vi "Temp_QCM_MKS_SNRaman.vi"() -> ()   [LabVIEW 2013]
doc: "This example demonstrates temperature control and monitoring.\n\nNote:\nBefore start this VI is it necessary:\n\n- preconfigure some specific parameters that are not supported by this driver (e.g. PV-I/O Type, Linearization type, Alarm Input Values... ) by Quick Codes, or by Eurotherm iTools or by instrument front panel controls\n- enter correct VISA Resource Descriptor, Device Address and Baud Rate into front-panel controls"
uses:
  LabVIEW Drivers for DVS instruments/_mks/common/mks pressure units.ctl
  LabVIEW Drivers for DVS instruments/_mks/common/mks status.ctl
  LabVIEW Drivers for DVS instruments/_mks/common/mks status control mode.ctl
  LabVIEW Drivers for DVS instruments/_mks/common/mks status learning mode.ctl
  LabVIEW Drivers for DVS instruments/_mks/common/mks status selection mode.ctl
  LabVIEW Drivers for DVS instruments/_mks/common/mks control direction.ctl
  LabVIEW Drivers for DVS instruments/_mks/common/mks setup communication mode.ctl
  LabVIEW Drivers for DVS instruments/_mks/common/mks setup termination character.ctl
  LabVIEW Drivers for DVS instruments/_mks/common/mks setpoint type.ctl
  LabVIEW Drivers for DVS instruments/_mks/common/mks control type.ctl
  <vilib>/Utility/file.llb/Write To Spreadsheet File (string).vi
  SpectraWiz_LV82_rev04Oct10-1chan-free.llb.llb/StellarNet SpectraWiz Globals.vi
  <instrlib>/Eurotherm 32xx Series/Eurotherm 32xx Series.lvlib
panel:
  in  "Stop SpectraNet Raman":bool
  in  "stop":bool
  in  "Tab Control":T1(tab)
  in  "Add comments to the data file here and click outside the comment box to submit.\nThe time at which comments are submitted is saved in the data file.":string
  out "New ALARM !":bool
  in  "Acknowledge All Alarms":bool
  in  "Controller  Mode":u8(ring) items=["Auto", "Manual"]
  in  "Temp Setpoint (C)":i16(slide)=25 min=0 max=1300 scale=0.0..500.0
  out "Temperature (C)":sgl
  out "Process Value - Chart":sgl(graph)
  in  "Keylock":u8(ring) items=["None", "All", "Edit", "mod", "mAn", "Stby", "tmr"]
  out "Alarm Output":bool
  in  "Alarm \nNumber (1)":u16=1 min=1 max=4
  out "Freq and Resistance Graph":T2(graph)
  out "pressure units 3":T3
  out "Waveform Chart 2":dbl(graph)
  out "status 2":T4
  out "Pressure 2":dbl
  in  "Control direction 3":T8
  in  "Setpoint 2":dbl(knob) min=0.0 max=100.0 scale=0.0..100.0
  out "Control direction 4":T8
  in  "Tab Control 2":T9(tab)=enum."Controls"
  in  "Channel to monitor":i8=1 min=1 max=1
  out "?":T10(graph)
  in  "Use Dark":bool
  in  "Channel":u8=1 min=1 max=1
  in  "Operating Parameters":T11(array[cluster]) {"Digitizer Clock Rate Setting" min=1 max=3; "Optical Smoothing Level" min=0 max=4 step=1; "Number of Scans to Average" min=1 max=10000 step=1}
  in  "Take Dark":bool
  in  "Take Reference":bool
  in  "Mode Selection":u16(ring) items=["Scope Mode", "Absorbance Mode", "Transmission Mode", "Radiometer Mode"]
  in  "View Data File":bool
  in  "Open Data File":bool
  out "?":T10(graph)
  in  "Reset Coefficients":bool
  in  "Drift Correct":bool
  in  "View Snapshot":bool
  in  "Take Snapshot":bool
  out "Number of Channels:":i32
  in  "Clear History":bool
  out "?":T10(graph)
  in  "Create and Log to Time Series Log File":bool
  out "ChartView":T12(graph)
  out "Cursor Indices":i32[](array[numeric])
  out "Data File":cluster{dbl[], dbl[]}
  out "Error Out":errorcluster
  out "Time [s]":dbl format="%.2f"
  # "Configuring Instrument\n \nPlease Wait......\n\nChart will update in 20 sec"
  # "Instructions:\n\nMake sure all instruments are plugged into the correct ports, the correct port numbers are set, and all instruments are turned on. \n\nTo begin, click the RUN arrow on the toolbar, and wait 20 seconds for instruments to begin recording.\n\nTo end, click \"END DATA LOGGING\" and \"Stop Spectra Raman\". DO NOT press the STOP button on the toolbar."
  # "© 2005-2010 StellarNet, Inc.,  All Right Reserved"
  # "``"
  # "© 2005-2013 StellarNet, Inc.,  All Right Reserved"
  # "© 2005-2010 StellarNet, Inc.,  All Right Reserved"
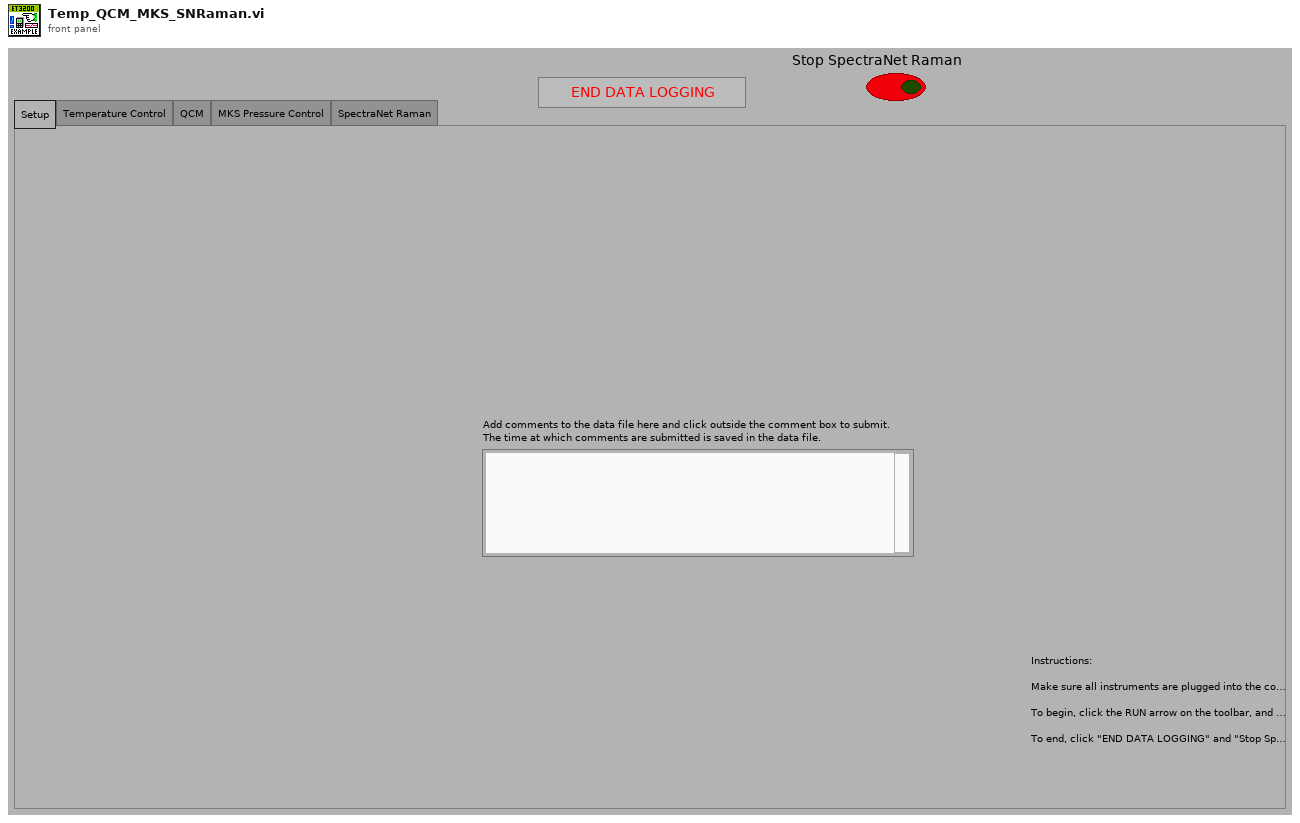
[diagram p1: front panel]
types:
  T1 = enum32{"Setup", "Temperature Control", "QCM", "MKS Pressure Control", "SpectraNet Raman"}
  T2 = cluster{"XY chart data":cluster{"x":dbl, "y":dbl}[]}[]
  T3 = typedef "mks pressure units.ctl" = enum16{"Torr", "mTorr", "mbar", "ubar", "kPa", "Pa", "cmH2O", "inH2O"}
  T4 = typedef "mks status.ctl" = cluster{"control mode":T5, "learning mode":T6, "selection mode":T7}
  T5 = typedef "mks status control mode.ctl" = enum16{"local", "remote"}
  T6 = typedef "mks status learning mode.ctl" = enum16{"not learning", "learning system", "learning valve"}
  T7 = typedef "mks status selection mode.ctl" = enum16{"open", "close", "stop", "setpoint A", "setpoint B", "setpoint C", "setpoint D", "setpoint E", "analog setpoint"}
  T8 = typedef "mks control direction.ctl" = enum16{"direct", "reverse"}
  T9 = enum32{"Graphical Display", "Controls", "Time Series"}
  T10 = cluster{"Spectrometer Wavelengths":dbl[], dbl[]}[]
  T11 = cluster{"Integration Time (ms)":i32, "Number of Scans to Average":i32, "Optical Smoothing Level":i32, "Digitizer Clock Rate Setting":i32, "Temp  Compensation ":bool}[]
  T12 = cluster{"Cursor Y":dbl, "Cursor Y":dbl, "Cursor Y":dbl}
  T13 = typedef "mks setup termination character.ctl" = enum16{"CRLF", "CR"}
  T14 = typedef "mks setup communication mode.ctl" = enum16{"8 databits no parity", "7 databits even parity"}
  T15 = cluster{"Cursor Y":dbl, "Cursor Y":dbl, "Cursor Y":dbl}[]
  T16 = cluster{"Coefficients":ext[], "Wavelengths":dbl[]}[]
  T17 = cluster{"[0]":dbl, "[1]":dbl, "[2]":dbl, "[3]":dbl, "[4]":dbl, "[5]":dbl, "[6]":dbl, "[7]":dbl, "[8]":dbl}
  T18 = cluster{"Minimum":dbl, "Maximum":dbl, "Increment":dbl, "Minor Incr":dbl, "Start":dbl}
  T19 = cluster{"Integration Time (ms)":i32, "Number of Scans to Average":i32, "Optical Smoothing Level":i32, "Digitizer Clock Rate Setting":i32, "Temp  Compensation ":bool}
  T20 = typedef "mks control type.ctl" = enum16{"Self-Tuning", "PID"}
  T21 = typedef "mks setpoint type.ctl" = enum16{"position", "pressure"}
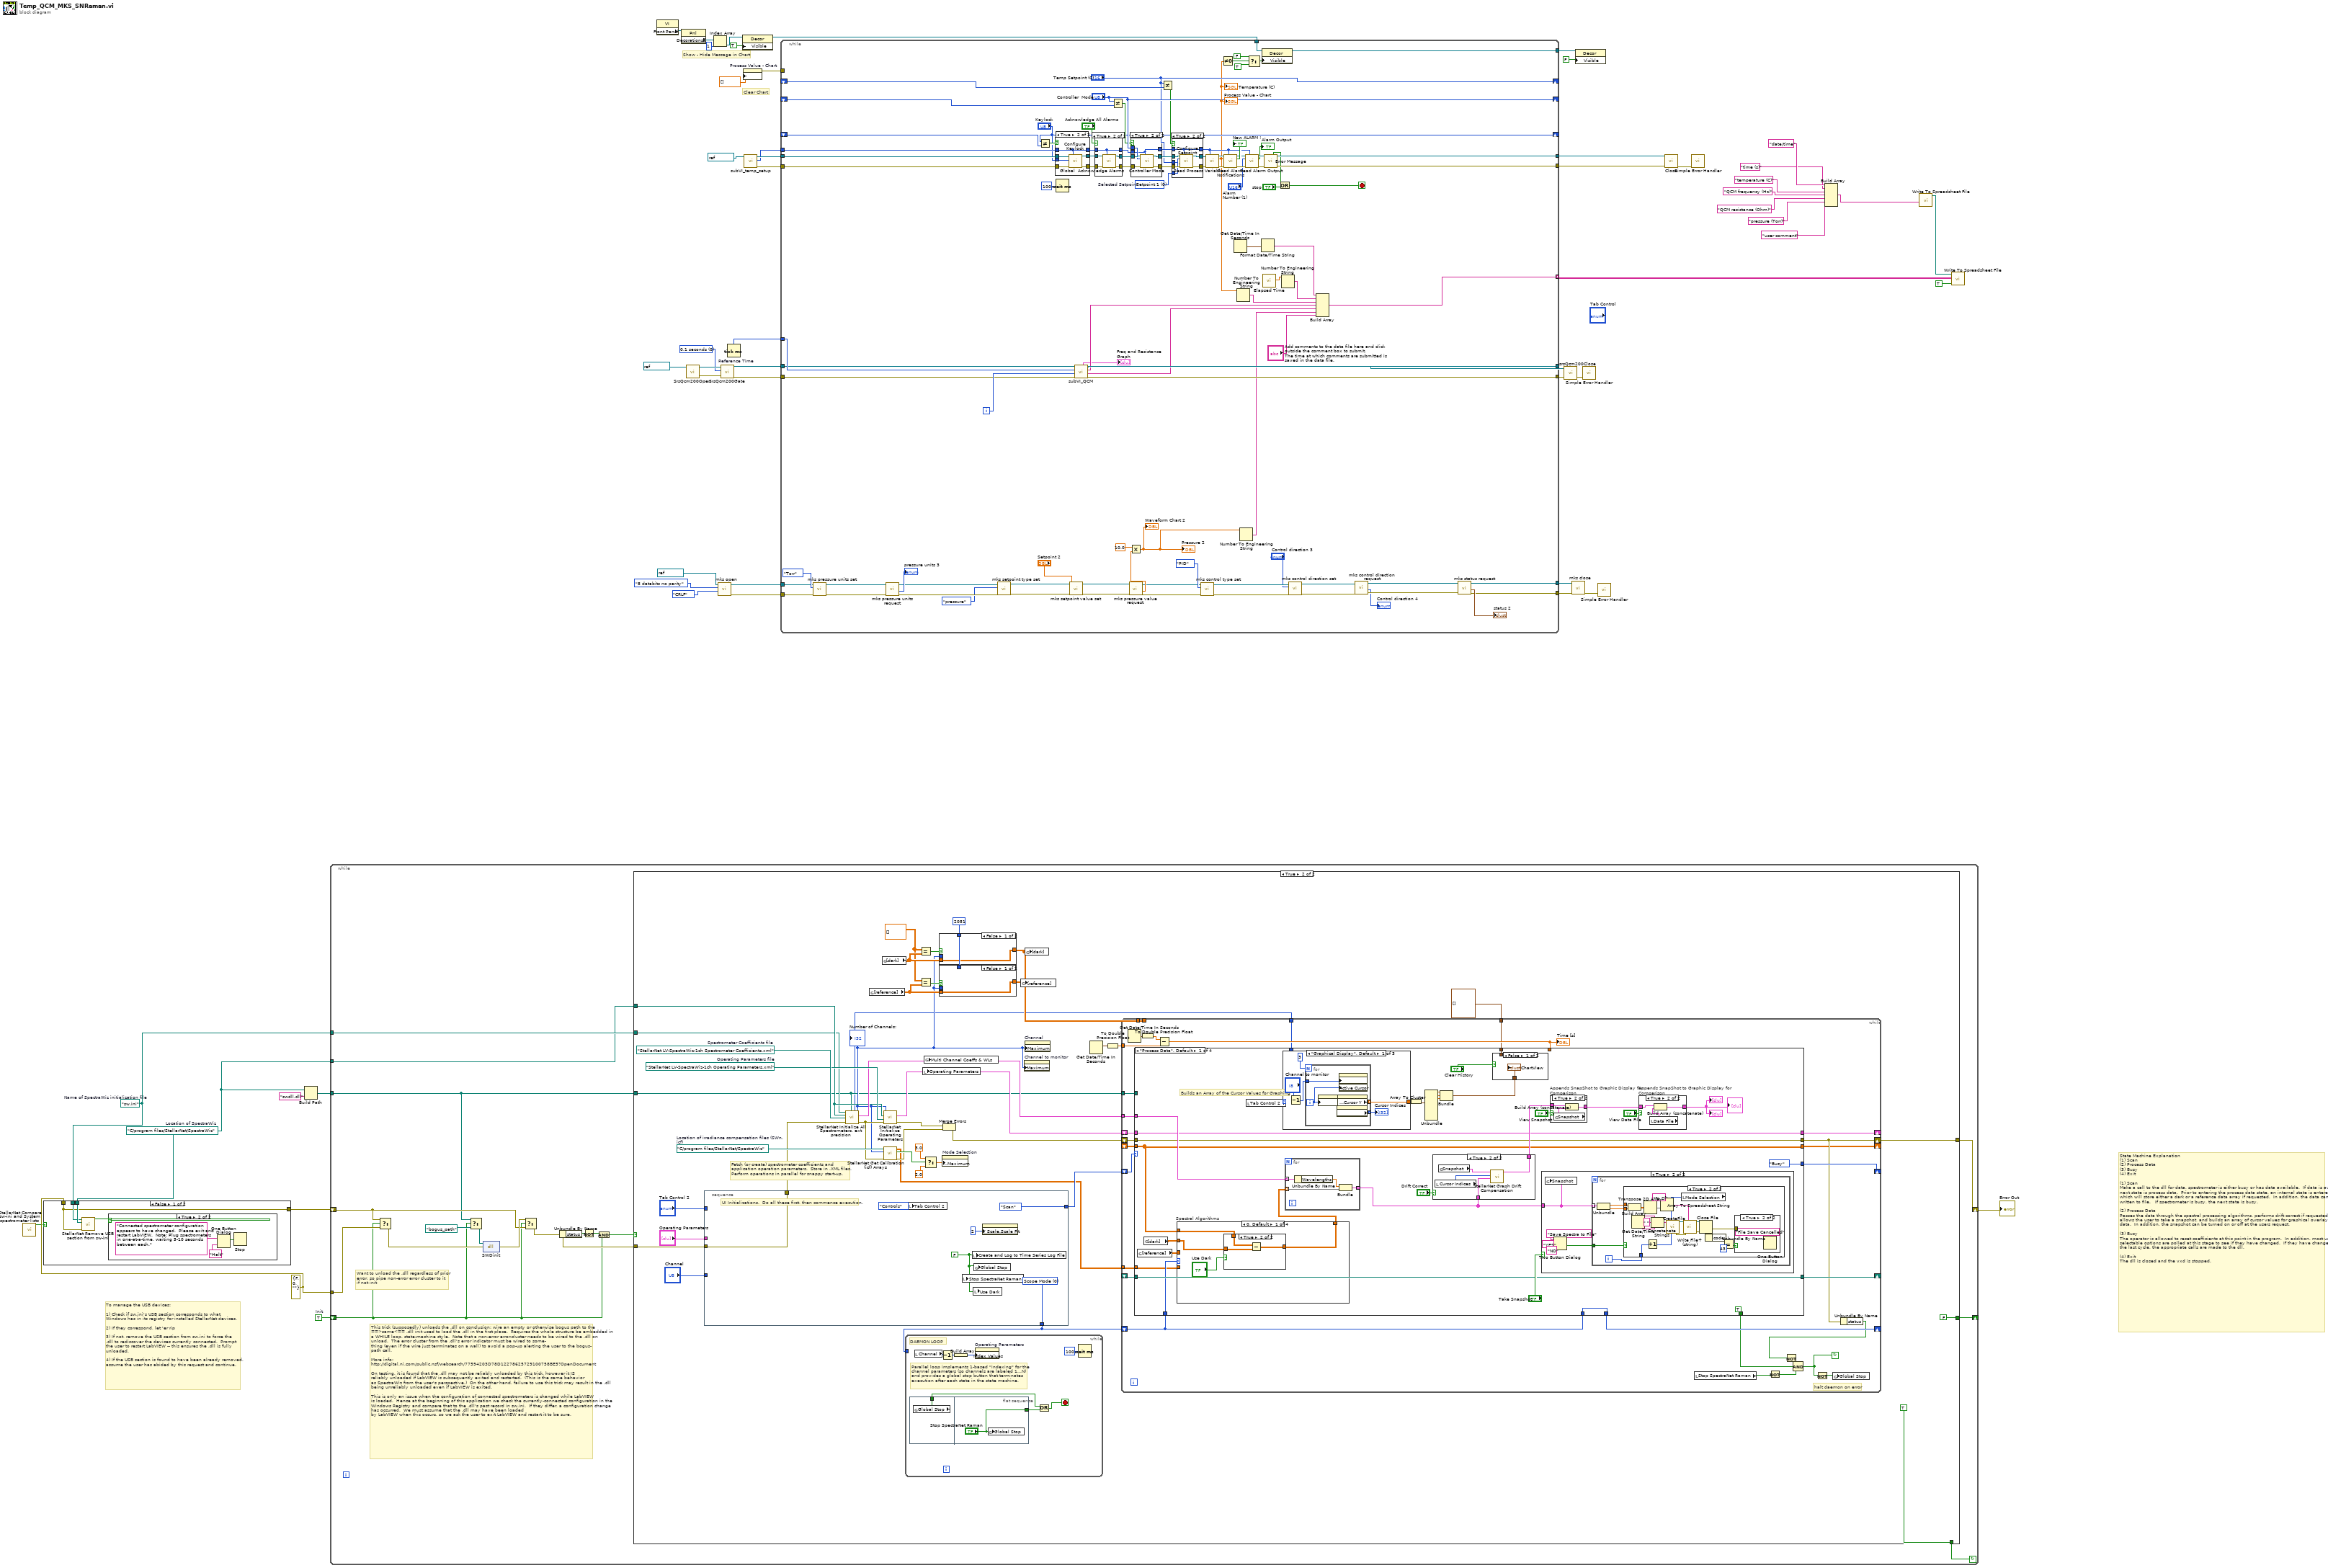
[diagram p0: block diagram]
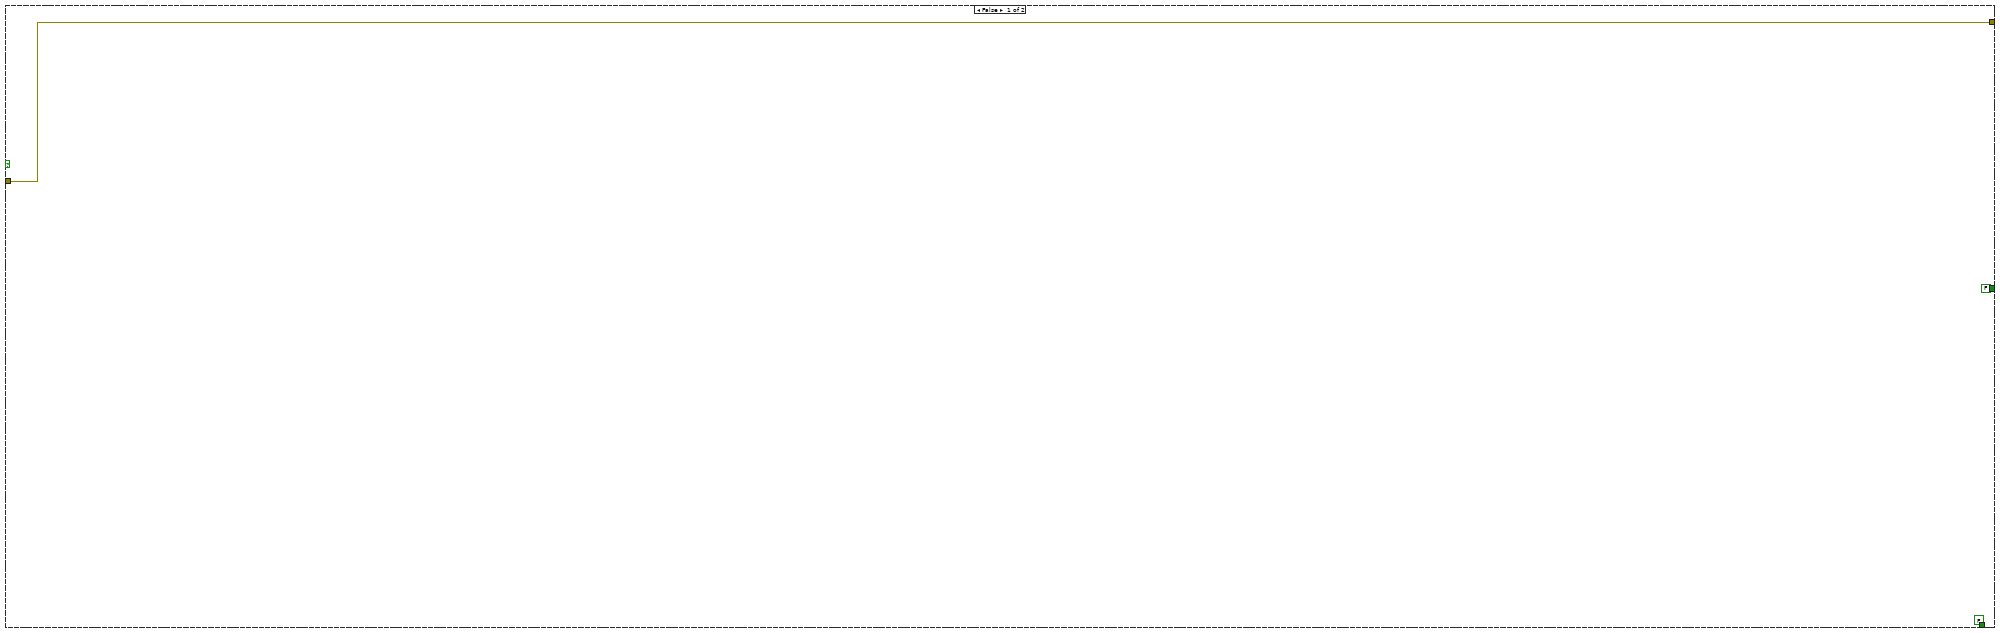
[diagram p4: hidden frame]
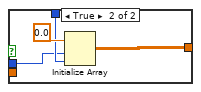
[diagram p5: hidden frame]
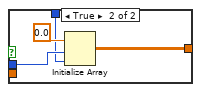
[diagram p6: hidden frame]
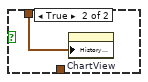
[diagram p7: hidden frame]
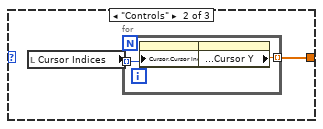
[diagram p8: hidden frame]
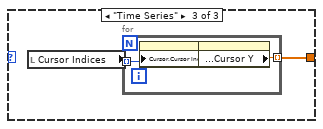
[diagram p9: hidden frame]
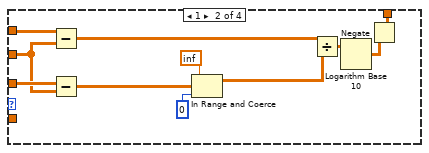
[diagram p14: hidden frame]
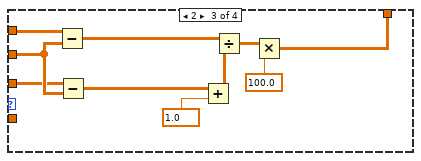
[diagram p15: hidden frame]
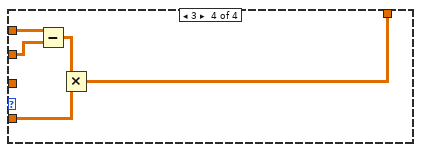
[diagram p16: hidden frame]
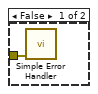
[diagram p19: hidden frame]
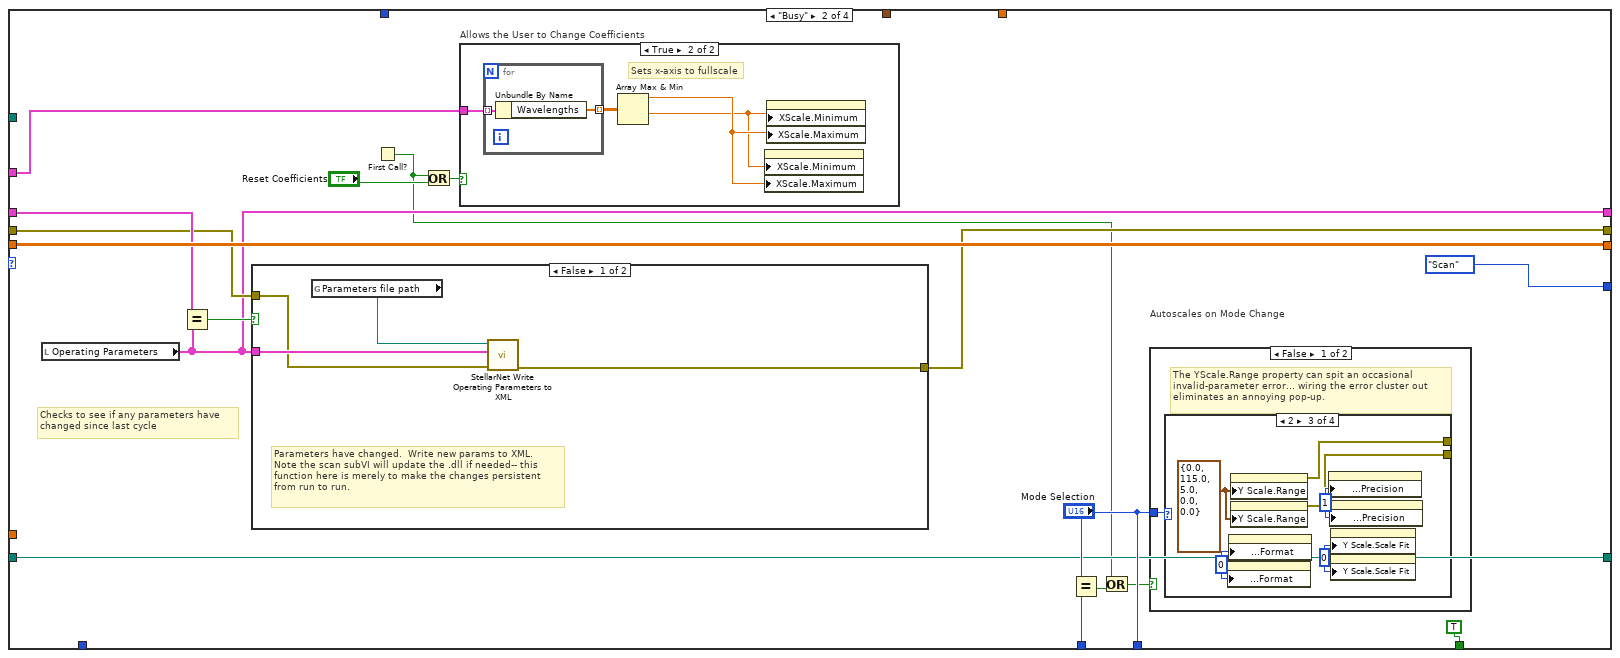
[diagram p20: hidden frame]
diagram:
  w5 = path "C:/program files/StellarNet/SpectraWiz"  # Location of SpectraWiz
  w10 = path "sw.ini"  # Name of SpectraWiz initialization file
  w7 = errorcluster {"status"=FALSE, "code"=0, "source"=""} ("error in (no error)")
  w11 = TRUE  # Init
  w30 = u16 0 items=["0.1 seconds", "1.0 seconds", "10.0 seconds"] ("Gate in")
  # "To manage the USB devices:\n\n1) Check if sw.ini's USB section corresponds to what\nWindows has in its registry for installed StellarNet devices.\n\n2) If they correspond, let 'er rip\n\n3) If not, remove the USB section from sw.ini to force the \n.dll to rediscover the devices currently connected.  Prompt\nthe user to restart LabVIEW -- this ensures the .dll is fully\nunloaded.  \n\n4) If the USB section is found to have been already removed, \nassume the user has abided by this request and continue."
  # "State Machine Explanation\n(1) Scan\n(2) Process Data\n(3) Busy\n(4) Exit\n\n(1) Scan\nMake a call to the dll for data, spectrometer is either busy or has data available.  If data is available, next state is process data.  Prior to entering the process data state, an internal state is entered which will store either a dark or a reference data array if requested.  In addition, the data can be written to file.   If spectrometer is busy, the next state is busy.\n\n(2) Process Data\nPasses the data through the spectral processing algorithms, performs drift correct if requested, allows the user to take a snapshot, and builds an array of cursor values for graphical overlay on the data.  In addition, the snapshot can be turned on or off at the users request.\n\n(3) Busy\nThe operator is allowed to reset coefficients at this point in the program.  In addition, most user selectable options are polled at this stage to see if they have changed.  If they have changed since the last cycle, the appropriate calls are made to the dll.\n\n(4) Exit\nThe dll is closed and the vxd is stopped."
  # "Show - Hide Message in Chart"
  # "Clear Chart"
  n1 = call "StellarNet Compare sw-ini and System spectrometer lists.vi"() -> ("Configs\nAgree"=w6:bool)  [unwired: 11 in]
  n2 = case shown="False" w6 {
    tunnel: w7 -> [w57 w63]
    tunnel: w5 -> [w59 _]
    tunnel: w10 -> [w58 _]
    tunnel: [w57 w63] -> w9
    frame False {
      n3 = call "StellarNet Remove USB section from sw-ini.vi"("error in (no error)"=w57, "Location of SpectraWiz"=w59, "Name of SpectraWiz initialization file"=w58) -> ("USB section found?"=w56:bool)  [unwired: 7 in, 1 out]
      n4 = case shown="True" w56 {
        frame False {
        }
        frame True {
          n5 = One Button Dialog(message="Connected spectrometer configuration appears to have changed.  Please exit and restart LabVIEW.  Note: Plug spectrometers in one-at-a-time, waiting 5-10 seconds between each.", button name ("OK")="Halt") -> (true=w61:bool)
          n6 = Stop(stop? (T)=w61) -> ()
        }
      }
    }
    frame True {
    }
  }
  n7 = Build Path(base path=w5, name or relative path="swdll.dll") -> (appended path=w3:path)
  n8 = while {
    shift-right: [w80] -> _
    shift-left: w11 -> [w66]
    tunnel: w10 -> [w73]
    tunnel: w5 -> [w65]
    shift-right: [w72] -> w8
    shift-left: w9 -> [w67]
    tunnel: w7 -> [w71]
    tunnel: w3 -> [w64]
    stop <- w79 continue-if-true
    # "This trick (supposedly) unloads the .dll on conclusion: wire an empty or otherwise bogus path to the ==>same<== .dll init used to load the .dll in the first place.  Requires the whole structure be embedded in a WHILE loop, state-machine style.  Note that a non-error error-cluster needs to be wired to the .dll on unload.  The error cluster from the .dll's error indicator must be wired to some-\nthing (even if the wire just terrminates on a wall) to avoid a pop-up alerting the user to the bogus-\npath call.\n\nMore info:\nhttp://digital.ni.com/public.nsf/websearch/77594203D78D12278625729100758BE5?OpenDocument\n\nOn testing, it is found that the .dll may not be reliably unloaded by this trick, however it IS\nreliably unloaded if LabVIEW is subsequently exited and restarted.  (This is the same behavior\nas SpectraWiz from the user's perspective.)  On the other hand, failure to use this trick may result in the .dll being unreliably unloaded even if LabVIEW is exited.\n\nThis is only an issue when the configuration of connected spectrometers is changed while LabVIEW\nis loaded.  Hence at the beginning of this application we check the currently-connected configuration in the Windows Registry and compare that to the .dll's past record in sw.ini.  If they differ, a configuration change has occurred.  We must assume that the .dll may have been loaded \nby LabVIEW when this occurs, so we ask the user to exit LabVIEW and restart it to be sure."
    # "Want to unload the .dll regardless of prior\nerror, so pipe non-error error cluster to it\nif not init"
    n9 = Select(t=w67, s=w66, f=w71) -> (s? t:f=w70:errorcluster)
    n10 = Select(t=w64, s=w66, f=path "bogus_path" ("reference")) -> (s? t:f=w77:path)
    n11 = dll-call lib="C:/Program Files/StellarNet/SpectraWiz/swdll.dll" fn="SWDinit" label="init"(path in=w77, error in=w70) -> (error out=w69:errorcluster)  [unwired: 2 in, 1 out]
    n12 = Select(t=w69, s=w66, f=w67) -> (s? t:f=w68:errorcluster)
    n13 = Unbundle By Name(w68) -> ("status"=w75:bool)
    n14 = Not(x=w75) -> (.not. x?=w76:bool)
    n15 = And(x=w76, y=w66) -> (x .and. y?=w74:bool)
    n16 = case shown="True" w74 {
      tunnel: [w81 w88] -> w72
      tunnel: w68 -> [w81 w94]
      tunnel: [FALSE ("Init") FALSE ("Init")] -> w80
      tunnel: [FALSE TRUE] -> w79
      tunnel: w65 -> [_ w90]
      tunnel: w73 -> [_ w89]
      tunnel: w64 -> [_ w85]
      frame False {
      }
      frame True {
        w95 = 2051 ("dimension size")
        w100 = sgl[][] [] ("[dark]")
        w119 = path "C:/program files/StellarNet/SpectraWiz"  # Location of irradiance compensation files (SWn.icf)
        w120 = path "StellarNet LV-SpectraWiz-1ch Operating Parameters.xml"  # Operating Parameters file
        w121 = path "StellarNet LV-SpectraWiz-1ch Spectrometer Coefficients.xml"  # Spectrometer Coefficients file
        # "Fetch (or create) spectrometer coefficients and\napplication operation parameters.  Store in .XML files.\nPerform operations in parallel for snappy start-up."
        n17 = stacked-sequence {
          tunnel: [w147] -> w103
          tunnel: [enum16{"Process Data", "Busy", "Exit", "Scan"}."Scan" ("Enum")] -> w111
          tunnel: "Tab Control 2" -> [_]
          tunnel: [w144] -> w91
          tunnel: "Channel" -> [_]
          tunnel: "Operating Parameters" -> [_]
          tunnel: w94 -> [w144]
          frame #0 {
            w147 = u16 0 items=["Scope Mode", "Absorbance Mode", "Transmission Mode", "Radiometer Mode"] ("Mode Selection")
            w143 = FALSE ("File Stamp")
            # "UI Initializations.  Do all these first, then commence execution."
            n18 = local write "Tab Control 2"(T9."Controls" ("Tab Control")) -> ()
            n19 = local write "Stop SpectraNet Raman"(w143) -> ()
            n20 = local write "Create and Log to Time Series Log File"(w143) -> ()
            n21 = local write "Use Dark"(w143) -> ()
            n22 = global write "StellarNet SpectraWiz Globals.vi" "Global Stop"(w143) -> ()
            n23 = property class="XYGraph (strict)"("Y Scale.Scale Fit"=u8 2) -> ()  [unwired: 2 in, 2 out]
          }
        }
        n24 = call "StellarNet Initialize All Spectrometers, ext precision.vi"("Path of swdll.dll"=w85, "error in"=w91, "Spectrometer Coefficients file"=w121, "Location of SpectraWiz"=w90, "Name of SpectraWiz initialization file"=w89) -> ("error out"=w118:errorcluster, "Multi Channel Coeffs & WLs"=w104:T16, "Number of Channels"=w86:i32, "Detector Types"=w84:u16[])  [unwired: 2 in, 1 out]
        "Number of Channels:" <- w86
        n25 = global read "StellarNet SpectraWiz Globals.vi" "[reference]"() -> (w98:sgl[][])
        n26 = global read "StellarNet SpectraWiz Globals.vi" "[dark]"() -> (w101:sgl[][])
        n27 = call "StellarNet Initialize Operating Parameters.vi"("error in"=w118, "Spectrometer Coefficients file"=w120, "Location of SpectraWiz"=w90, "Number of Channels"=w86) -> ("error out"=w113:errorcluster, "Operating Parameters"=w108:T11)  [unwired: 6 in]
        n28 = call "StellarNet Get Calibration (icf) Arrays.vi"("error in (no error)"=w118, "Number of Channels"=w86, "directory path"=w119) -> ("error out"=w112:errorcluster, ".icf found for\nat least one channel"=w114:bool, "N x Compensation Array"=w109:dbl[][])  [unwired: 6 in]
        n29 = while {
          tunnel: w103 -> [_]
          stop <- w134 stop-if-true
          # "DAEMON LOOP"
          # "Parallel loop implements 1-based \"indexing\" for the \nchannel parameters (so channels are labeled 1...N)\nand provides a global stop button that terminates\nexecution after each state in the state machine."
          n30 = flat-sequence {
            tunnel: [w141] -> w136
            tunnel: ["Stop SpectraNet Raman"] -> w135
            frame #0 {
              n31 = global read "StellarNet SpectraWiz Globals.vi" "Global Stop"() -> (w141:bool)
            }
            frame #1 {
              n32 = global write "StellarNet SpectraWiz Globals.vi" "Global Stop"("Stop SpectraNet Raman") -> ()
            }
          }
          n33 = local read "Channel"() -> (w139:u8)
          n34 = Decrement(x=w139) -> (x-1=w138:u8)
          n35 = Build Array(w138) -> (w137:u8[])
          n36 = property on="Operating Parameters" class="Arr (strict)"("Index Values"=w137) -> ()  [unwired: 2 in, 2 out]
          n37 = Or(x=w136, y=w135) -> (x .or. y?=w134:bool)
          n38 = Wait (ms)(milliseconds to wait=u32 100) -> ()  [unwired: 1 out]
        }
        n39 = Equal?(x=w100, y=w101) -> (x = y?=w102:bool)
        n40 = Equal?(x=w100, y=w98) -> (x = y?=w99:bool)
        n41 = local write "Operating Parameters"(w108) -> ()
        n42 = global write "StellarNet SpectraWiz Globals.vi" "Multi Channel Coeffs & WLs"(w104) -> ()
        n43 = Select(t=3.0 ("Data Range:Maximum"), s=w114, f=2.0 ("Data Range:Maximum")) -> (s? t:f=w117:dbl)
        n44 = case shown="False" w102 {
          tunnel: [w129 w133] -> w97
          tunnel: w101 -> [w129 _]
          tunnel: w86 -> [_ w131]
          tunnel: w95 -> [_ w130]
          frame False {
          }
          frame True {
            n45 = Initialize Array(0.0, w131, w130) -> (w133:dbl[][])
          }
        }
        n46 = case shown="False" w99 {
          tunnel: [w124 w128] -> w96
          tunnel: w98 -> [w124 _]
          tunnel: w86 -> [_ w125]
          tunnel: w95 -> [_ w126]
          frame False {
          }
          frame True {
            n47 = Initialize Array(0.0, w125, w126) -> (w128:dbl[][])
          }
        }
        n48 = property on="Mode Selection" class="Ring (strict)"("Data Range:Maximum"=w117) -> ()  [unwired: 2 in, 2 out]
        n49 = Merge Errors(w113, w112) -> (w110:errorcluster)
        n50 = global write "StellarNet SpectraWiz Globals.vi" "[reference]"(w96) -> ()
        n51 = property on="Channel to monitor" class="DigNum (strict)"("Maximum"=w86) -> ()  [unwired: 2 in, 2 out]
        n52 = property on="Channel" class="DigNum (strict)"("Maximum"=w86) -> ()  [unwired: 2 in, 2 out]
        n53 = global write "StellarNet SpectraWiz Globals.vi" "[dark]"(w97) -> ()
        n54 = Get Date/Time In Seconds() -> (seconds since 1Jan1904=w122:timestamp)
        n55 = To Double Precision Float(number=w122) -> (double precision float=w123:dbl)
        n56 = while {
          tunnel: w123 -> [w175]
          shift-right: [w174] -> _
          shift-left: w103 -> [w167]
          shift-right: [w172] -> _
          shift-left: w111 -> [w173]
          shift-right: [w169] -> _
          shift-left: _ -> [w170]
          shift-right: [w165] -> w88
          shift-left: w110 -> [w166]
          shift-right: [w164] -> _
          shift-left: _ -> [w163]
          tunnel: w104 -> [w162]
          tunnel: w109 -> [w161]
          tunnel: w97 -> [_]
          tunnel: w96 -> [_]
          shift-right: [w152] -> _
          shift-left: w108 -> [w160]
          tunnel: T15 [] ("History Data") -> [w151]
          tunnel: w85 -> [w150]
          tunnel: w84 -> [w149]
          stop <- w156 continue-if-true
          # "halt daemon on error"
          n57 = Get Date/Time In Seconds() -> (seconds since 1Jan1904=w168:timestamp)
          n58 = To Double Precision Float(number=w168) -> (double precision float=w176:dbl)
          n59 = Subtract(x=w176, y=w175) -> (x-y=w171:dbl)
          "Time [s]" <- w171
          n60 = case shown="\"Process Data\", Default" w173 {
            tunnel: w167 -> [w199 w329 w373 w395]
            tunnel: [w199 "Mode Selection" w373 w395] -> w174
            tunnel: [enum16{"Process Data", "Busy", "Exit", "Scan"}."Busy" ("Enum") enum16{"Process Data", "Busy", "Exit", "Scan"}."Scan" ("Enum") enum16{"Process Data", "Busy", "Exit", "Scan"}."Process Data" ("Enum") enum16{"Process Data", "Busy", "Exit", "Scan"}."Process Data" ("Enum")] -> w172
            tunnel: [TRUE TRUE FALSE TRUE] -> w157
            tunnel: [w186 w323 w368 w382] -> w164
            tunnel: w171 -> [_ _ _ w403]
            tunnel: w170 -> [w194 w325 w371 w404]
            tunnel: [w194 w325 w371 w402] -> w169
            tunnel: w167 -> [w193 _ _ _]
            tunnel: w160 -> [w180 w322 w366 w387]
            tunnel: w166 -> [w181 w320 w367 w384]
            tunnel: [w181 w319 w367 w389] -> w165
            tunnel: w163 -> [w186 w323 w368 _]
            tunnel: w162 -> [w187 w324 _ _]
            tunnel: w161 -> [w184 _ _ _]
            tunnel: [w180 w318 w366 w387] -> w152
            tunnel: w151 -> [w178 _ _ _]
            tunnel: w150 -> [_ _ _ w383]
            tunnel: w149 -> [_ _ _ w378]
            frame "Process Data", Default {
              # "Builds an Array of the Cursor Values for Graphing"
              n61 = global read "StellarNet SpectraWiz Globals.vi" "[reference]"() -> (w188:sgl[][])
              n62 = global read "StellarNet SpectraWiz Globals.vi" "[dark]"() -> (w189:sgl[][])
              n63 = case "Spectral Algorithms" shown="0, Default" w193 {
                tunnel: [w249 w263 w271 w277] -> w185
                tunnel: w186 -> [w248 w262 w268 w279]
                tunnel: w189 -> [w247 w258 w266 w276]
                tunnel: w188 -> [_ w259 w265 _]
                tunnel: w184 -> [_ _ _ w275]
                frame 0, Default {
                  n64 = case shown="True" "Use Dark" {
                    tunnel: [w250 w253] -> w249
                    tunnel: w248 -> [w250 w252]
                    tunnel: w247 -> [_ w251]
                    frame False {
                    }
                    frame True {
                      n65 = Subtract(x=w252, y=w251) -> (x-y=w253:sgl[][])
                    }
                  }
                }
                frame 1 {
                  n66 = Subtract(x=w262, y=w258) -> (x-y=w261:sgl[][])
                  n67 = Subtract(x=w259, y=w258) -> (x-y=w255:sgl[][])
                  n68 = In Range and Coerce(upper limit=inf, x=w255, lower limit=0) -> (coerced(x)=w254:dbl[][])  [unwired: 1 out]
                  n69 = Divide(x=w261, y=w254) -> (x/y=w260:dbl[][])
                  n70 = Logarithm Base 10(1:w260) -> (0:w264:dbl[][])
                  n71 = Negate(x=w264) -> (-x=w263:dbl[][])
                }
                frame 2 {
                  n72 = Subtract(x=w268, y=w266) -> (x-y=w274:sgl[][])
                  n73 = Subtract(x=w265, y=w266) -> (x-y=w269:sgl[][])
                  n74 = Add(x=w269, y=sgl 1.0) -> (x+y=w267:sgl[][])
                  n75 = Divide(x=w274, y=w267) -> (x/y=w273:sgl[][])
                  n76 = Multiply(x=w273, y=sgl 100.0) -> (x*y=w271:sgl[][])
                }
                frame 3 {
                  n77 = Subtract(x=w279, y=w276) -> (x-y=w278:sgl[][])
                  n78 = Multiply(x=w278, y=w275) -> (x*y=w277:dbl[][])
                }
              }
              n79 = local read "Tab Control 2"() -> (w191:T9)
              n80 = case shown="\"Graphical Display\", Default" w191 {
                tunnel: [w216 w224 w228] -> w204
                frame "Graphical Display", Default {
                  n81 = Decrement(x="Channel to monitor") -> (x-1=w213:i8)
                  n82 = for {
                    N: 3 -> [_]
                    tunnel: [w222] -> w216 mode=indexing
                    tunnel: [w220] -> w215 mode=indexing
                    tunnel: w213 -> [w218]
                    i -> [w219]
                    n83 = property class="XYGraph (strict)"("Active Cursor"=w219) -> (error out=w221:errorcluster)  [unwired: 2 in, 1 out]
                    n84 = property class="XYGraph (strict)"(error in=w221) -> ("Cursor.Cursor Index"=w220:i32)  [unwired: 1 in, 2 out]
                    n85 = property class="XYGraph (strict)"(error in=w221) -> ("Cursor.Cursor Position:Cursor Y"=w222:dbl)  [unwired: 1 in, 2 out]
                    n86 = property class="XYGraph (strict)"("Cursor.Cursor Plot"=w218, "Active Cursor"=w219) -> ()  [unwired: 2 in, 2 out]
                  }
                  "Cursor Indices" <- w215
                }
                frame "Controls" {
                  n87 = local read "Cursor Indices"() -> (w223:i32[])
                  n88 = for {
                    tunnel: [w227] -> w224 mode=indexing
                    tunnel: w223 -> [w225] mode=indexing
                    n89 = property class="XYGraph (strict)"("Cursor.Cursor Index"=w225) -> (error out=w226:errorcluster)  [unwired: 2 in, 1 out]
                    n90 = property class="XYGraph (strict)"(error in=w226) -> ("Cursor.Cursor Position:Cursor Y"=w227:dbl)  [unwired: 1 in, 2 out]
                  }
                }
                frame "Time Series" {
                  n91 = local read "Cursor Indices"() -> (w229:i32[])
                  n92 = for {
                    tunnel: [w232] -> w228 mode=indexing
                    tunnel: w229 -> [w230] mode=indexing
                    n93 = property class="XYGraph (strict)"("Cursor.Cursor Index"=w230) -> (error out=w231:errorcluster)  [unwired: 2 in, 1 out]
                    n94 = property class="XYGraph (strict)"(error in=w231) -> ("Cursor.Cursor Position:Cursor Y"=w232:dbl)  [unwired: 1 in, 2 out]
                  }
                }
              }
              n95 = for {
                tunnel: w187 -> [w212] mode=indexing
                tunnel: w185 -> [w210] mode=indexing
                tunnel: [w209] -> w183 mode=indexing
                n96 = Unbundle By Name(w212) -> ("Wavelengths"=w211:dbl[])
                n97 = Bundle("Wavelengths"=w211, w210) -> (w209:cluster{"Wavelengths":dbl[], dbl[]})  [unwired: 1 in]
              }
              n98 = Array To Cluster(array=w204) -> (cluster=w203:T17)
              n99 = Unbundle(w203) -> ("[0]"=w202:dbl, "[1]"=w201:dbl, "[2]"=w200:dbl)  [unwired: 6 out]
              n100 = case shown="True" "Drift Correct" {
                tunnel: w183 -> [w237 w241]
                tunnel: [w237 w238] -> w196
                frame False {
                }
                frame True {
                  n101 = local read "Cursor Indices"() -> (w239:i32[])
                  n102 = global read "StellarNet SpectraWiz Globals.vi" "Snapshot"() -> (w240:cluster{"Wavelengths":dbl[], sgl[]}[])
                  n103 = call "StellarNet Graph Drift Compensation.vi"("Current Graph"=w241, "Cursor Indices"=w239, "Snapshot"=w240) -> ("De-Drifted Current Graph"=w238:cluster{"Wavelengths":dbl[], sgl[]}[])  [unwired: 8 in]
                }
              }
              n104 = Bundle("[0]"=w202, "[1]"=w201, "[2]"=w200) -> (w177:cluster{"[0]":dbl, "[1]":dbl, "[2]":dbl})  [unwired: 1 in]
              n105 = case shown="False" "Clear History" {
                tunnel: w178 -> [_ w208]
                tunnel: w177 -> [w207 _]
                frame False {
                  "ChartView" <- w207
                }
                frame True {
                  n106 = property on="ChartView" class="WFChart (strict)"("History Data"=w208) -> ()  [unwired: 2 in, 2 out]
                }
              }
              n107 = case shown="True" "Take Snapshot" {
                tunnel: w183 -> [_ w280]
                frame False {
                }
                frame True {
                  n108 = global write "StellarNet SpectraWiz Globals.vi" "Snapshot"(w280) -> ()
                  n109 = Two Button Dialog(message="Save Spectra to File", 1:"NO" ("F button name (\"Cancel\")"), 2:"YES" ("T button name (\"OK\")")) -> (T button?=w284:bool)
                  n110 = for {
                    tunnel: w284 -> [w289]
                    tunnel: w280 -> [w288] mode=indexing
                    i -> [w285]
                    n111 = Unbundle(w288) -> ("Wavelengths"=w287:dbl[], w286:dbl[])
                    n112 = case shown="True" w289 {
                      tunnel: w287 -> [_ w300]
                      tunnel: w286 -> [_ w299]
                      tunnel: w285 -> [_ w291]
                      frame False {
                      }
                      frame True {
                        n113 = Build Array(w300, w299) -> (w293:dbl[][])
                        n114 = Get Date/Time String() -> (date string=w306:string, time string=w305:string)  [unwired: 3 in]
                        n115 = Transpose 2D Array(2D array=w293) -> (transposed array=w301:dbl[][])
                        n116 = Increment(x=w291) -> (x+1=w290:i32)
                        n117 = Concatenate Strings(w306, " ", w305) -> (w307:string)
                        n118 = Array To Spreadsheet String(array=w301, 3:"%.2f" ("format string")) -> (spreadsheet string=w302:string)  [unwired: 1 in]
                        n119 = local read "Mode Selection"() -> (w292:u16)
                        n120 = call "CreateFile.vi"("Time Stamp"=w307, "Mode Selection"=w292, "Channel (1-based)"=w290) -> ("Refnumber"=w309:refnum<file>, "Error Out"=w308:errorcluster)  [unwired: 2 in, 2 out]
                        n121 = call <vilib>:"Write File+ (string).vi"("string"=w302, "error in (no error)"=w308, "refnum"=w309) -> ("error out"=w298:errorcluster, "dup refnum"=w310:refnum<file>)  [unwired: 4 in, 1 out]
                        n122 = Close File(refnum=w310, error in=w298) -> (error out=w294:errorcluster)  [unwired: 1 out]
                        n123 = Unbundle By Name(w294) -> ("code"=w296:i32)
                        n124 = Equal?(x=w296, y=43) -> (x = y?=w295:bool)
                        n125 = case shown="True" w295 {
                          tunnel: w294 -> [w311 _]
                          frame False {
                            n126 = call <vilib>:"Simple Error Handler.vi"("error in (no error)"=w311) -> ()  [unwired: 4 in, 5 out]
                          }
                          frame True {
                            n127 = One Button Dialog(message="File Save Cancelled") -> ()  [unwired: 1 in, 1 out]
                          }
                        }
                      }
                    }
                  }
                }
              }
              n128 = case "Appends SnapShot to Graphic Display for Comparison" shown="True" "View Snapshot" {
                tunnel: w196 -> [w242 w245]
                tunnel: [w242 w243] -> w182
                frame False {
                }
                frame True {
                  n129 = global read "StellarNet SpectraWiz Globals.vi" "Snapshot"() -> (w244:cluster{"Wavelengths":dbl[], sgl[]}[])
                  n130 = Build Array (concatenate)(w245, w244) -> (w243:cluster{"Wavelengths":dbl[], dbl[]}[])
                }
              }
              n131 = case "Appends SnapShot to Graphic Display for Comparison" shown="True" "View Data File" {
                tunnel: w182 -> [w233 w236]
                tunnel: [w233 w234] -> w190
                frame False {
                }
                frame True {
                  n132 = local read "Data File"() -> (w235:cluster{dbl[], dbl[]})
                  n133 = Build Array (concatenate)(w236, w235) -> (w234:cluster{"Wavelengths":dbl[], dbl[]}[])
                }
              }
              "?" <- w190
              "?" <- w190
              "?" <- w190
            }
            frame "Busy" {
              # "Checks to see if any parameters have \nchanged since last cycle"
              n134 = local read "Operating Parameters"() -> (w318:T11)
              n135 = Equal?(x=w322, y=w318) -> (x = y?=w321:bool)
              n136 = case shown="False" w321 {
                tunnel: w318 -> [w332 _]
                tunnel: w320 -> [w331 w334]
                tunnel: [w330 w334] -> w319
                frame False {
                  # "Parameters have changed.  Write new params to XML.\nNote the scan subVI will update the .dll if needed-- this\nfunction here is merely to make the changes persistent\nfrom run to run."
                  n137 = global read "StellarNet SpectraWiz Globals.vi" "Parameters file path"() -> (w333:path)
                  n138 = call "StellarNet Write Operating Parameters to XML.vi"("error in (no error)"=w331, "Operating Parameters"=w332, "XML File Path"=w333) -> ("error out"=w330:errorcluster)  [unwired: 8 in]
                }
                frame True {
                  # "Parameters are the same.  Do nothing."
                }
              }
              n139 = First Call?() -> (First Call?: T/F=w314:bool)
              n140 = Or(x=w314, y="Reset Coefficients") -> (x .or. y?=w316:bool)
              n141 = case "Allows the User to Change Coefficients" shown="True" w316 {
                tunnel: w324 -> [_ w363]
                frame False {
                }
                frame True {
                  # "Sets x-axis to fullscale"
                  n142 = for {
                    tunnel: w363 -> [w365] mode=indexing
                    tunnel: [w364] -> w362 mode=indexing
                    n143 = Unbundle By Name(w365) -> ("Wavelengths"=w364:dbl[])
                  }
                  n144 = Array Max & Min(array=w362) -> (max value=w361:dbl, min value=w360:dbl)  [unwired: 2 out]
                  n145 = property class="XYGraph (strict)"("XScale.Minimum"=w360, "XScale.Maximum"=w361) -> ()  [unwired: 2 in, 2 out]
                  n146 = property class="XYGraph (strict)"("XScale.Minimum"=w360, "XScale.Maximum"=w361) -> ()  [unwired: 2 in, 2 out]
                }
              }
              n147 = Equal?(x="Mode Selection", y=w329) -> (x = y?=w315:bool)
              n148 = Or(x=w314, y=w315) -> (x .or. y?=w313:bool)
              n149 = case "Autoscales on Mode Change" shown="False" w313 {
                tunnel: "Mode Selection" -> [w335 _]
                frame False {
                  # "The YScale.Range property can spit an occasional \ninvalid-parameter error... wiring the error cluster out \neliminates an annoying pop-up."
                  n150 = case shown="2" w335 {
                    tunnel: [w337 w343 w349 w355] -> _
                    tunnel: [w336 w342 w348 w354] -> _
                    frame 0, Default {
                      w338 = 0
                      w339 = T18 {"Minimum"=0.0, "Maximum"=4096.0, "Increment"=1000.0, "Minor Incr"=100.0, "Start"=0.0} ("Y Scale.Range")
                      w341 = 0
                      w340 = u8 0 ("Y Scale.Scale Fit")
                      n151 = property class="XYGraph (strict)"("Y Scale.Range"=w339) -> (error out=w336:errorcluster)  [unwired: 2 in, 1 out]
                      n152 = property class="XYGraph (strict)"("Y Scale.Range"=w339) -> (error out=w337:errorcluster)  [unwired: 2 in, 1 out]
                      n153 = property class="XYGraph (strict)"("Y Scale.Format & Precision:Format"=w338) -> ()  [unwired: 2 in, 2 out]
                      n154 = property class="XYGraph (strict)"("Y Scale.Format & Precision:Format"=w338) -> ()  [unwired: 2 in, 2 out]
                      n155 = property class="XYGraph (strict)"("Y Scale.Format & Precision:Precision"=w341) -> ()  [unwired: 2 in, 2 out]
                      n156 = property class="XYGraph (strict)"("Y Scale.Format & Precision:Precision"=w341) -> ()  [unwired: 2 in, 2 out]
                      n157 = property class="XYGraph (strict)"("Y Scale.Scale Fit"=w340) -> ()  [unwired: 2 in, 2 out]
                      n158 = property class="XYGraph (strict)"("Y Scale.Scale Fit"=w340) -> ()  [unwired: 2 in, 2 out]
                    }
                    frame 1 {
                      w344 = 0
                      w347 = 1
                      w346 = T18 {"Minimum"=0.0, "Maximum"=3.0, "Increment"=0.001, "Minor Incr"=0.0, "Start"=0.0} ("Y Scale.Range")
                      w345 = u8 0 ("Y Scale.Scale Fit")
                      n159 = property class="XYGraph (strict)"("Y Scale.Range"=w346) -> (error out=w342:errorcluster)  [unwired: 2 in, 1 out]
                      n160 = property class="XYGraph (strict)"("Y Scale.Range"=w346) -> (error out=w343:errorcluster)  [unwired: 2 in, 1 out]
                      n161 = property class="XYGraph (strict)"("Y Scale.Format & Precision:Format"=w344) -> ()  [unwired: 2 in, 2 out]
                      n162 = property class="XYGraph (strict)"("Y Scale.Format & Precision:Format"=w344) -> ()  [unwired: 2 in, 2 out]
                      n163 = property class="XYGraph (strict)"("Y Scale.Format & Precision:Precision"=w347) -> ()  [unwired: 2 in, 2 out]
                      n164 = property class="XYGraph (strict)"("Y Scale.Format & Precision:Precision"=w347) -> ()  [unwired: 2 in, 2 out]
                      n165 = property class="XYGraph (strict)"("Y Scale.Scale Fit"=w345) -> ()  [unwired: 2 in, 2 out]
                      n166 = property class="XYGraph (strict)"("Y Scale.Scale Fit"=w345) -> ()  [unwired: 2 in, 2 out]
                    }
                    frame 2 {
                      w350 = T18 {"Minimum"=0.0, "Maximum"=115.0, "Increment"=5.0, "Minor Incr"=0.0, "Start"=0.0} ("Y Scale.Range")
                      w351 = 0
                      w353 = 1
                      w352 = u8 0 ("Y Scale.Scale Fit")
                      n167 = property class="XYGraph (strict)"("Y Scale.Format & Precision:Format"=w351) -> ()  [unwired: 2 in, 2 out]
                      n168 = property class="XYGraph (strict)"("Y Scale.Format & Precision:Format"=w351) -> ()  [unwired: 2 in, 2 out]
                      n169 = property class="XYGraph (strict)"("Y Scale.Range"=w350) -> (error out=w349:errorcluster)  [unwired: 2 in, 1 out]
                      n170 = property class="XYGraph (strict)"("Y Scale.Range"=w350) -> (error out=w348:errorcluster)  [unwired: 2 in, 1 out]
                      n171 = property class="XYGraph (strict)"("Y Scale.Format & Precision:Precision"=w353) -> ()  [unwired: 2 in, 2 out]
                      n172 = property class="XYGraph (strict)"("Y Scale.Format & Precision:Precision"=w353) -> ()  [unwired: 2 in, 2 out]
                      n173 = property class="XYGraph (strict)"("Y Scale.Scale Fit"=w352) -> ()  [unwired: 2 in, 2 out]
                      n174 = property class="XYGraph (strict)"("Y Scale.Scale Fit"=w352) -> ()  [unwired: 2 in, 2 out]
                    }
                    frame 3 {
                      w356 = 1
                      w357 = T18 {"Minimum"=0.0, "Maximum"=1.0, "Increment"=0.1, "Minor Incr"=0.01, "Start"=0.0} ("Y Scale.Range")
                      w359 = 2
                      w358 = u8 0 ("Y Scale.Scale Fit")
                      n175 = property class="XYGraph (strict)"("Y Scale.Range"=w357) -> (error out=w354:errorcluster)  [unwired: 2 in, 1 out]
                      n176 = property class="XYGraph (strict)"("Y Scale.Range"=w357) -> (error out=w355:errorcluster)  [unwired: 2 in, 1 out]
                      n177 = property class="XYGraph (strict)"("Y Scale.Format & Precision:Format"=w356) -> ()  [unwired: 2 in, 2 out]
                      n178 = property class="XYGraph (strict)"("Y Scale.Format & Precision:Format"=w356) -> ()  [unwired: 2 in, 2 out]
                      n179 = property class="XYGraph (strict)"("Y Scale.Format & Precision:Precision"=w359) -> ()  [unwired: 2 in, 2 out]
                      n180 = property class="XYGraph (strict)"("Y Scale.Format & Precision:Precision"=w359) -> ()  [unwired: 2 in, 2 out]
                      n181 = property class="XYGraph (strict)"("Y Scale.Scale Fit"=w358) -> ()  [unwired: 2 in, 2 out]
                      n182 = property class="XYGraph (strict)"("Y Scale.Scale Fit"=w358) -> ()  [unwired: 2 in, 2 out]
                    }
                  }
                }
                frame True {
                }
              }
            }
            frame "Exit" {
              n183 = local write "Create and Log to Time Series Log File"(FALSE ("File Stamp")) -> ()
            }
            frame "Scan" {
              # "Truncate return array for \nnumber of pixels in spectrum"
              n184 = case shown="False" "Open Data File" {
                frame False {
                }
                frame True {
                  n185 = call <vilib>:"Read Characters From File.vi"() -> ("character string"=w422:string)  [unwired: 6 in, 3 out]
                  n186 = Search and Replace String(replace all?=TRUE ("replace all? (F)"), input string=w422, search string="\r\n ", replace string="\r\n") -> (result string=w426:string)  [unwired: 4 in, 3 out]
                  n187 = Search and Replace String(replace all?=TRUE ("replace all? (F)"), input string=w426, search string="  ", replace string="\t") -> (result string=w430:string)  [unwired: 4 in, 3 out]
                  n188 = Spreadsheet String To Array(delimiter (Tab)="\t", format string="%f", spreadsheet string=w430) -> (array=w433:dbl[][])  [unwired: 1 in]
                  n189 = Transpose 2D Array(2D array=w433) -> (transposed array=w421:dbl[][])
                  n190 = Delete From Array(array=w421, index (col)=0 ("disabled index (col)")) -> (array with subset deleted=w418:dbl[][])  [unwired: 2 in, 1 out]
                  n191 = Delete From Array(array=w418, index (col)=0 ("disabled index (col)")) -> (array with subset deleted=w416:dbl[][])  [unwired: 2 in, 1 out]
                  n192 = Index Array(array=w416, index (row)=0) -> (element=w415:dbl[])  [unwired: 1 in]
                  n193 = Index Array(array=w416, index (row)=1) -> (element=w413:dbl[])  [unwired: 1 in]
                  n194 = Bundle(w415, w413) -> (→"Data File":cluster{dbl[], dbl[]})  [unwired: 1 in]
                }
              }
              n195 = local read "Channel"() -> (w379:u8)
              n196 = Decrement(x=w379) -> (x-1=w381:u8)
              n197 = Index Array(array=w387, index=w381) -> (element=w385:T19)
              n198 = Index Array(array=w378, index=w379) -> (element=w377:u16)
              n199 = case shown="5" w377 {
                tunnel: [2048 512 1024] -> w380
                frame 1, Default {
                }
                frame 5 {
                }
                frame 6 {
                }
              }
              n200 = Decrement(x=w380) -> (x-1=w376:i32)
              n201 = call "StellarNet Single-Channel Scan rev A.vi"("Path of sw.dll"=w383, "error in (no error)"=w384, "Operation Settings"=w385, "Channel (1-based)"=w379) -> ("error out"=w386:errorcluster, "buffer out"=w375:sgl[])  [unwired: 4 in, 2 out]
              n202 = Split 1D Array(array=w375, index=w376) -> (first subarray=w374:sgl[])  [unwired: 1 out]
              n203 = Build Array(w374) -> (w382:sgl[][])
              n204 = Build Array("Counts", "Absorbance (au)", "% Transmission", "Irradiance (Watts/m^2)") -> (w396:string[])
              n205 = Index Array(array=w396, index=w395) -> (element=w394:string)
              n206 = local read "ChartView"() -> (w391:T12)
              n207 = case "Populates  Reference Array" shown="True" "Take Reference" {
                tunnel: w382 -> [_ w411]
                frame False {
                }
                frame True {
                  n208 = global write "StellarNet SpectraWiz Globals.vi" "[reference]"(w411) -> ()
                }
              }
              n209 = case "Populates  Dark Array" shown="True" "Take Dark" {
                tunnel: w382 -> [_ w410]
                frame False {
                }
                frame True {
                  n210 = global write "StellarNet SpectraWiz Globals.vi" "[dark]"(w410) -> ()
                  n211 = local write "Use Dark"(TRUE ("Use Dark")) -> ()
                }
              }
              n212 = property class="XYGraph (strict)"("Y Scale.Name Label.Text"=w394) -> ()  [unwired: 2 in, 2 out]
              n213 = property class="XYGraph (strict)"("Y Scale.Name Label.Text"=w394) -> ()  [unwired: 2 in, 2 out]
              n214 = call "File Stamp.vi"("ChartView"=w391, "File Stamp"="Create and Log to Time Series Log File", "Time [s]"=w403, "Error In"=w386, "File Path In"=w404) -> ("File Path Out"=w402:path, "Error Out"=w389:errorcluster)  [unwired: 9 in]
            }
          }
          n215 = local read "Stop SpectraNet Raman"() -> (w154:bool)
          n216 = Not(x=w154) -> (.not. x?=w153:bool)
          n217 = Unbundle By Name(w165) -> ("status"=w159:bool)
          n218 = Not(x=w159) -> (.not. x?=w158:bool)
          n219 = Compound Arithmetic op=AND(w158, w157, w153) -> (w156:bool)
          n220 = Not(x=w156) -> (.not. x?=w155:bool)
          n221 = global write "StellarNet SpectraWiz Globals.vi" "Global Stop"(w155) -> ()
        }
      }
    }
  }
  "Error Out" <- w8
  n222 = property class="VI"() -> ("Front Panel"=w48:refnum<vi>)  [unwired: 2 in, 2 out]
  n223 = property class="Pnl"(reference=w48) -> ("Decorations[]"=w49:refnum<vi>[])  [unwired: 1 in, 2 out]
  n224 = call <instrlib>:"SrsQcm200Open.vi"("VISA in"=refnum<visa-resource-name> "COM6") -> ("error out"=w34:errorcluster, "VISA out"=w33:refnum<visa-resource-name>)  [unwired: 4 in]
  n225 = Index Array(array=w49, index=1) -> (element=w46:refnum<vi>)
  n226 = call "mks open.vi"("termination character"=mks_setup_termination_character."CRLF", "comm. mode"=mks_setup_communication_mode."8 databits no parity", "VISA in"=refnum<visa-resource-name> "COM5") -> ("error out"=w15:errorcluster, "VISA out"=w16:refnum<visa-resource-name>)  [unwired: 7 in]
  n227 = call <instrlib>:"SrsQcm200Gate.vi"("VISA in"=w33, "Gate in"=w30, "error in (no error)"=w34) -> ("VISA out"=w27:refnum<visa-resource-name>, "error out"=w26:errorcluster)  [unwired: 14 in, 1 out]
  n228 = Tick Count (ms) "Reference Time"() -> (millisecond timer value=w28:u32)
  n229 = property class="Decor"(reference=w46, "Visible"=TRUE) -> (reference out=w45:refnum<vi>)  [unwired: 1 in, 1 out]
  n230 = property on="Process Value - Chart" class="WFChart (strict)"("History Data"=sgl[] []) -> (error out=w41:errorcluster)  [unwired: 2 in, 1 out]
  n231 = call "subVI_temp_setup.vi"("VISA Refnum in"=refnum<visa-resource-name> "COM4" ("VISA resource name")) -> ("error out"=w54:errorcluster, "Unit Address (1)"=w35:u8, "VISA Refnum out"=w55:refnum<visa-resource-name>)  [unwired: 8 in]
  n232 = while {
    tunnel: w55 -> [w500]
    tunnel: w54 -> [w499]
    tunnel: w35 -> [w501]
    tunnel: [w521] -> w52
    tunnel: [w520] -> w53
    shift-right: ["Keylock"] -> _
    shift-left: _ -> [w510]
    shift-right: ["Controller  Mode"] -> _
    shift-left: _ -> [w507]
    shift-right: ["Temp Setpoint (C)"] -> _
    shift-left: _ -> [w505]
    tunnel: w45 -> [w485]
    tunnel: [w483] -> w43
    tunnel: w41 -> [_]
    tunnel: [w479] -> w29 mode=indexing
    tunnel: w28 -> [w477]
    tunnel: w27 -> [w476]
    tunnel: w26 -> [w475]
    tunnel: [w474] -> w25
    tunnel: [w473] -> w24
    tunnel: w16 -> [w443]
    tunnel: w15 -> [w442]
    tunnel: [w441] -> w13
    tunnel: [w440] -> w12
    i -> [w478]
    stop <- w514 stop-if-true
    w516 = u8 0 items=["Setpoint 1", "Setpoint 2", "Alternate Setpoint", "Target Setpoint"]  # Selected Setpoint
    n233 = call "mks pressure units set.vi"("error in (no error)"=w442, "pressure units"=mks_pressure_units."Torr", "VISA in"=w443) -> ("error out"=w456:errorcluster, "VISA out"=w455:refnum<visa-resource-name>)  [unwired: 7 in]
    n234 = call "mks pressure units request.vi"("error in (no error)"=w456, "VISA in"=w455) -> ("error out"=w458:errorcluster, "pressure units"=→"pressure units 3":T3, "VISA out"=w457:refnum<visa-resource-name>)  [unwired: 7 in]
    n235 = call "mks setpoint type set.vi"("error in (no error)"=w458, "setpoint type"=mks_setpoint_type."pressure", "VISA in"=w457) -> ("error out"=w446:errorcluster, "VISA out"=w445:refnum<visa-resource-name>)  [unwired: 7 in]
    n236 = Not Equal?(x="Keylock", y=w510) -> (x != y?=w509:bool)
    n237 = case shown="True" w509 {
      tunnel: w500 -> [w558 w565]
      tunnel: w499 -> [w557 w564]
      tunnel: [w558 w563] -> w529
      tunnel: [w557 w562] -> w528
      tunnel: w501 -> [w559 w561]
      tunnel: [w559 w561] -> w518
      tunnel: "Keylock" -> [_ w560]
      frame False {
      }
      frame True {
        n238 = call <instrlib>:"Configure Keylock.vi"("VISA resource name"=w565, "Unit Address (1)"=w561, "Keylock"=w560, "error in (no error)"=w564) -> ("VISA resource name out"=w563:refnum<visa-resource-name>, "error out"=w562:errorcluster)  [unwired: 10 in]
      }
    }
    n239 = Wait (ms)(milliseconds to wait=u32 100) -> ()  [unwired: 1 out]
    n240 = call "mks setpoint value set.vi"("error in (no error)"=w446, "setpoint"="Setpoint 2", "VISA in"=w445) -> ("error out"=w451:errorcluster, "VISA out"=w450:refnum<visa-resource-name>)  [unwired: 7 in]
    n241 = call "subVI_QCM.vi"("error in (no error)"=w475, "Loop iteration number"=w478, "millisecond timer value"=w477, "VISA Refnum in"=w476) -> ("error out"=w473:errorcluster, "Resistance (Ohm)"=w471:string, "Freq (Hz)"=w472:string, "VISA Refnum out"=w474:refnum<visa-resource-name>, "Freq and Resistance Graph"=→"Freq and Resistance Graph":T2)  [unwired: 3 in]
    n242 = case shown="True" "Acknowledge All Alarms" {
      tunnel: w529 -> [w550 w556]
      tunnel: w528 -> [w549 w555]
      tunnel: [w550 w554] -> w523
      tunnel: [w549 w553] -> w522
      tunnel: w518 -> [w551 w552]
      tunnel: [w551 w552] -> w517
      frame False {
      }
      frame True {
        n243 = call <instrlib>:"Global  Acknowledge Alarms.vi"("VISA resource name"=w556, "Unit Address (1)"=w552, "error in (no error)"=w555) -> ("VISA resource name out"=w554:refnum<visa-resource-name>, "error out"=w553:errorcluster)  [unwired: 11 in]
      }
    }
    n244 = Not Equal?(x="Controller  Mode", y=w507) -> (x != y?=w506:bool)
    n245 = call "mks pressure value request.vi"("error in (no error)"=w451, "VISA in"=w450) -> ("error out"=w453:errorcluster, "pressure"=w468:dbl, "VISA out"=w452:refnum<visa-resource-name>)  [unwired: 7 in]
    n246 = Multiply(x=10.0, y=w468) -> (x*y=w439:dbl)
    "Pressure 2" <- w439
    "Waveform Chart 2" <- w439
    n247 = case shown="True" w506 {
      tunnel: [w540 w548] -> w527
      tunnel: [w541 w547] -> w524
      tunnel: w523 -> [w541 w546]
      tunnel: w522 -> [w540 w545]
      tunnel: w517 -> [w542 w543]
      tunnel: "Controller  Mode" -> [_ w544]
      tunnel: [w542 w543] -> w515
      frame False {
      }
      frame True {
        n248 = call <instrlib>:"Controller Mode.vi"("VISA resource name"=w546, "Unit Address (1)"=w543, "Controller Mode (0: Auto)"=w544, "error in (no error)"=w545) -> ("VISA resource name out"=w547:refnum<visa-resource-name>, "error out"=w548:errorcluster)  [unwired: 10 in]
      }
    }
    n249 = Not Equal?(x="Temp Setpoint (C)", y=w505) -> (x != y?=w503:bool)
    n250 = case shown="True" w503 {
      tunnel: w527 -> [w530 w539]
      tunnel: [w530 w538] -> w526
      tunnel: [w531 w537] -> w525
      tunnel: w524 -> [w531 w536]
      tunnel: w516 -> [_ w535]
      tunnel: w515 -> [w532 w534]
      tunnel: [w532 w534] -> w490
      tunnel: "Temp Setpoint (C)" -> [_ w533]
      frame False {
      }
      frame True {
        n251 = call <instrlib>:"Configure Setpoint.vi"("VISA resource name"=w536, "Unit Address (1)"=w534, "Setpoint (0: Setpoint 1)"=w535, "Setpoint Value (0)"=w533, "error in (no error)"=w539) -> ("VISA resource name out"=w537:refnum<visa-resource-name>, "error out"=w538:errorcluster)  [unwired: 9 in]
      }
    }
    n252 = call "mks control type set.vi"("error in (no error)"=w453, "control type"=mks_control_type."PID", "VISA in"=w452) -> ("error out"=w463:errorcluster, "VISA out"=w462:refnum<visa-resource-name>)  [unwired: 7 in]
    n253 = call <instrlib>:"Read Process Variables.vi"("VISA resource name"=w525, "Unit Address (1)"=w490, "error in (no error)"=w526) -> ("VISA resource name out"=w498:refnum<visa-resource-name>, "Process Value"=w481:sgl, "error out"=w497:errorcluster)  [unwired: 9 in, 1 out]
    "Temperature (C)" <- w481
    "Process Value - Chart" <- w481
    n254 = Not Equal To 0?(x=w481) -> (x != 0?=w486:bool)
    n255 = call <instrlib>:"Read Alarm Notifications.vi"("VISA resource name"=w498, "Unit Address (1)"=w490, "error in (no error)"=w497) -> ("VISA resource name out"=w494:refnum<visa-resource-name>, "New Alarm"=→"New ALARM !":bool, "error out"=w495:errorcluster)  [unwired: 10 in]
    n256 = Get Date/Time In Seconds() -> (seconds since 1Jan1904=w482:timestamp)
    n257 = Number To Engineering String(4:w481) -> (0:w480:string)  [unwired: 3 in]
    n258 = Number To Engineering String(4:w439) -> (0:w438:string)  [unwired: 3 in]
    n259 = call <instrlib>:"Read Alarm Output.vi"("VISA resource name"=w494, "Unit Address (1)"=w490, "Alarm Number (1)"="Alarm \nNumber (1)", "error in (no error)"=w495) -> ("VISA resource name out"=w493:refnum<visa-resource-name>, "Alarm Output"=→"Alarm Output":bool, "error out"=w492:errorcluster)  [unwired: 9 in]
    n260 = Select(t=FALSE ("Visible"), s=w486, f=TRUE ("Visible")) -> (s? t:f=w488:bool)
    n261 = Format Date/Time String(seconds (now)=w482) -> (date/time string=w435:string)  [unwired: 2 in]
    n262 = property class="Decor"(reference=w485, "Visible"=w488) -> (reference out=w483:refnum<vi>)  [unwired: 1 in, 1 out]
    n263 = call "Elapsed Time"() -> ("Elapsed Time (s)"=w436:dbl)  [unwired: 12 in, 7 out]
    n264 = call <instrlib>:"Error Message.vi"("VISA resource name"=w493, "error in (no error)"=w492) -> ("Status"=w512:bool, "VISA resource name out"=w521:refnum<visa-resource-name>, "error out"=w520:errorcluster)  [unwired: 9 in, 2 out]
    n265 = Or(x=w512, y="stop") -> (x .or. y?=w514:bool)
    n266 = Number To Engineering String(4:w436) -> (0:w434:string)  [unwired: 3 in]
    n267 = call "mks control direction set.vi"("error in (no error)"=w463, "direction"="Control direction 3", "VISA in"=w462) -> ("error out"=w464:errorcluster, "VISA out"=w465:refnum<visa-resource-name>)  [unwired: 7 in]
    n268 = Build Array(w435, w434, w480, w472, w471, w438, "Add comments to the data file here and click outside the comment box to submit.\nThe time at which comments are submitted is saved in the data file.") -> (w479:string[])
    n269 = call "mks control direction request.vi"("error in (no error)"=w464, "VISA in"=w465) -> ("error out"=w461:errorcluster, "direction"=→"Control direction 4":T8, "VISA out"=w460:refnum<visa-resource-name>)  [unwired: 7 in]
    n270 = call "mks status request.vi"("error in (no error)"=w461, "VISA in"=w460) -> ("error out"=w440:errorcluster, "status"=→"status 2":T4, "VISA out"=w441:refnum<visa-resource-name>)  [unwired: 7 in]
  }
  n271 = call <instrlib>:"srsQcm200Close.vi"("error in"=w24, "Visa in"=w25) -> ("error out"=w31:errorcluster)  [unwired: 3 in]
  n272 = call "mks close.vi"("error in (no error)"=w12, "VISA in"=w13) -> ("error out"=w14:errorcluster)  [unwired: 9 in]
  n273 = property class="Decor"(reference=w43, "Visible"=FALSE) -> ()  [unwired: 1 in, 2 out]
  n274 = call <vilib>:"Simple Error Handler.vi"("error in (no error)"=w31) -> ()  [unwired: 4 in, 5 out]
  n275 = call <vilib>:"Simple Error Handler.vi"("error in (no error)"=w14) -> ()  [unwired: 4 in, 5 out]
  n276 = call <instrlib>:"Close.vi"("VISA resource name"=w52, "error in (no error)"=w53) -> ("error out"=w51:errorcluster)  [unwired: 13 in]
  n277 = call <vilib>:"Simple Error Handler.vi"("error in (no error)"=w51) -> ()  [unwired: 4 in, 5 out]
  n278 = Build Array("date/time", "time (s)", "temperature (C)", "QCM frequency (Hz)", "QCM resistance (Ohm)" ("element"), "pressure (Torr)" ("element"), "user comment" ("element")) -> (w38:string[])
  n279 = call-poly <vilib>:"Write To Spreadsheet File.vi"("1D data"=w38) -> ("new file path (Not A Path if cancelled)"=w37:path)  [unwired: 7 in]
  n280 = call-poly <vilib>:"Write To Spreadsheet File.vi"("append to file? (new file:F)"=TRUE, "2D data"=w29, "file path (dialog if empty)"=w37) -> ()  [unwired: 5 in, 1 out]
